vi "Update Map File Path.vi"(8 "error in (no error)":errorcluster, 10 "Map File Path":path, 11 "Map Model in":refnum<class "Map Model.lvclass">) -> (0 "error out":errorcluster, 3 "Map Model out":refnum<class "Map Model.lvclass">)   [LabVIEW 2020, in "Map Model.lvlib" / "Map Model.lvclass"]
uses:
  Map Model.lvclass
  <vilib>/Utility/miscctls.llb/LVPointTypeDef.ctl
  Map Model.lvclass/Map Model.ctl
  Stack/Stack.lvclass
panel:
  # "NOTICE -- YOU MUST LEAVE THIS NOTICE IN PLACE.\n\nCopyright (c) 2017, LIANG LIU Shawn.Liu.cn@gmail.com\nAll rights reserved.\n\nRedistribution and use in source and binary forms, with or without modification, are permitted provided that the following conditions are met:\n-Redistributions of source code must retain the above copyright notice, this list of conditions and the following disclaimer.\n-Redistributions in binary form must reproduce the above copyright notice, this list of conditions and the following disclaimer in the documentation and/or other materials provided with the distribution.\n-Neither the name of the eLp nor the names of its contributors may be used to endorse or promote products derived from this software without specific prior written permission.\n\nTHIS SOFTWARE IS PROVIDED BY THE COPYRIGHT HOLDERS AND CONTRIBUTORS \"AS IS\" AND ANY EXPRESS OR IMPLIED WARRANTIES, INCLUDING, BUT NOT LIMITED TO, THE IMPLIED WARRANTIES OF MERCHANTABILITY AND FITNESS FOR A PARTICULAR PURPOSE ARE DISCLAIMED. IN NO EVENT SHALL THE COPYRIGHT HOLDER OR CONTRIBUTORS BE LIABLE FOR ANY DIRECT, INDIRECT, INCIDENTAL, SPECIAL, EXEMPLARY, OR CONSEQUENTIAL DAMAGES (INCLUDING, BUT NOT LIMITED TO, PROCUREMENT OF SUBSTITUTE GOODS OR SERVICES; LOSS OF USE, DATA, OR PROFITS; OR BUSINESS INTERRUPTION) HOWEVER CAUSED AND ON ANY THEORY OF LIABILITY, WHETHER IN CONTRACT, STRICT LIABILITY, OR TORT (INCLUDING NEGLIGENCE OR OTHERWISE) ARISING IN ANY WAY OUT OF THE USE OF THIS SOFTWARE, EVEN IF ADVISED OF THE POSSIBILITY OF SUCH DAMAGE."
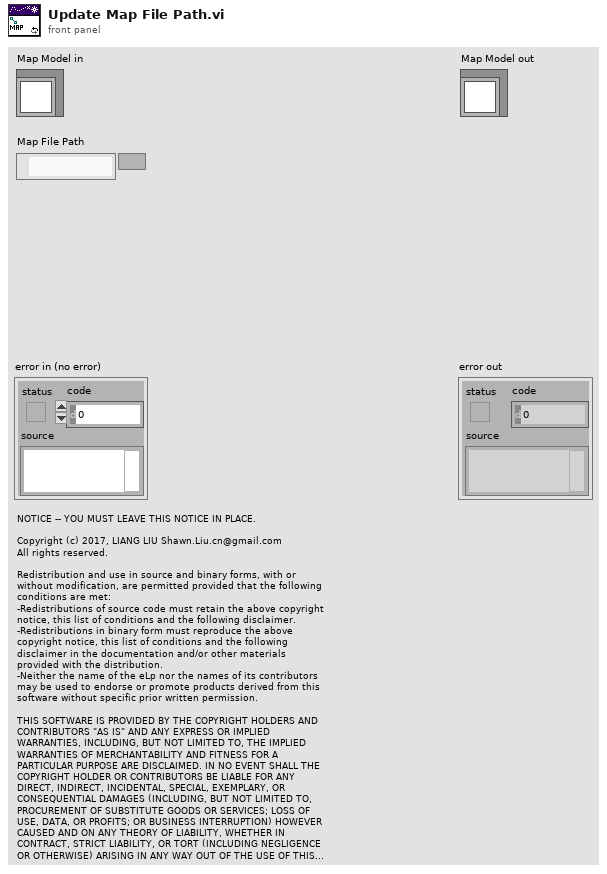
[diagram p1: front panel]
types:
  T1 = typedef "LVPointTypeDef.ctl" = cluster{"Horizontal":i16, "Vertical":i16}
  T2 = enum8{"Enabled", "Disabled", "Disabled and Grayed Out"}
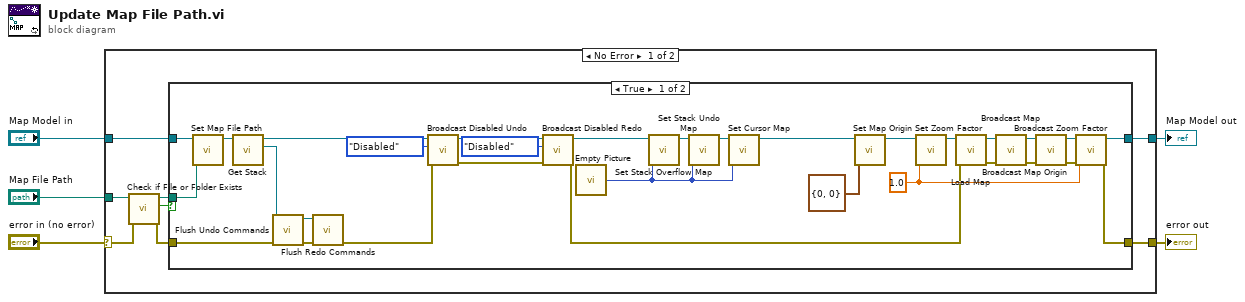
[diagram p0: block diagram]
diagram:
  n1 = case shown="No Error" "error in (no error)" {
    selector: "error in (no error)" -> [w9 w48]
    tunnel: "Map Model in" -> [w13 w47]
    tunnel: [w12 w48] -> w4
    tunnel: [w11 w47] -> w3
    tunnel: "Map File Path" -> [w10 _]
    frame No Error {
      n2 = call <vilib>:"Check if File or Folder Exists.vi"("error in (no error)"=w9, "path"=w10) -> ("error out"=w6:errorcluster, "file or folder exists?"=w7:bool, "dup path"=w8:path)  [unwired: 7 in]
      n3 = case shown="True" w7 {
        tunnel: w13 -> [w44 w46]
        tunnel: [w15 w45] -> w12
        tunnel: [w20 w46] -> w11
        tunnel: w8 -> [w43 _]
        tunnel: w6 -> [w27 w45]
        frame True {
          w19 = 1.0 ("Zoom Factor")
          n4 = call "Set Map File Path.vi"("Map File Path"=w43, "Map Model in"=w44) -> ("Map Model out"=w29:refnum<class "Map Model.lvclass">)  [unwired: 9 in]
          n5 = call "Get Stack.vi"("Map Model in"=w29) -> ("Stack"=w28:refnum<class "Stack.lvclass">, "Map Model out"=w32:refnum<class "Map Model.lvclass">)  [unwired: 9 in]
          n6 = call "Flush Undo Commands.vi"("error in (no error)"=w27, "Stack in"=w28) -> ("error out"=w37:errorcluster, "Stack out"=w36:refnum<class "Stack.lvclass">)  [unwired: 8 in]
          n7 = call "Flush Redo Commands.vi"("error in (no error)"=w37, "Stack in"=w36) -> ("error out"=w30:errorcluster)  [unwired: 8 in, 1 out]
          n8 = call "Broadcast Disabled Undo.vi"("error in (no error)"=w30, "Disabled Undo"=T2."Disabled", "Map Model in"=w32) -> ("error out"=w31:errorcluster, "Map Model out"=w35:refnum<class "Map Model.lvclass">)  [unwired: 7 in]
          n9 = call "Broadcast Disabled Redo.vi"("error in (no error)"=w31, "Disabled Redo"=T2."Disabled", "Map Model in"=w35) -> ("error out"=w18:errorcluster, "Map Model out"=w14:refnum<class "Map Model.lvclass">)  [unwired: 7 in]
          n10 = call "Empty Picture"() -> ("empty picture"=w38:picture)
          n11 = call "Set Stack Overflow Map.vi"("Stack Overflow Map"=w38, "Map Model in"=w14) -> ("Map Model out"=w40:refnum<class "Map Model.lvclass">)  [unwired: 9 in]
          n12 = call "Set Stack Undo Map.vi"("Stack Undo Map"=w38, "Map Model in"=w40) -> ("Map Model out"=w39:refnum<class "Map Model.lvclass">)  [unwired: 9 in]
          n13 = call "Set Cursor Map.vi"("Cursor Map"=w38, "Map Model in"=w39) -> ("Map Model out"=w26:refnum<class "Map Model.lvclass">)  [unwired: 9 in]
          n14 = call "Set Map Origin.vi"("Map Origin"=T1 {"Horizontal"=0, "Vertical"=0}, "Map Model in"=w26) -> ("Map Model out"=w25:refnum<class "Map Model.lvclass">)  [unwired: 9 in]
          n15 = call "Set Zoom Factor.vi"("Zoom Factor"=w19, "Map Model in"=w25) -> ("Map Model out"=w24:refnum<class "Map Model.lvclass">)  [unwired: 9 in]
          n16 = call "Load Map.vi"("error in (no error)"=w18, "Map Model in"=w24) -> ("error out"=w41:errorcluster, "Map Model out"=w42:refnum<class "Map Model.lvclass">)  [unwired: 8 in]
          n17 = call "Broadcast Map.vi"("error in (no error)"=w41, "Map Model in"=w42) -> ("error out"=w17:errorcluster, "Map Model out"=w23:refnum<class "Map Model.lvclass">)  [unwired: 8 in]
          n18 = call "Broadcast Map Origin.vi"("error in (no error)"=w17, "Map Model in"=w23) -> ("error out"=w16:errorcluster, "Map Model out"=w22:refnum<class "Map Model.lvclass">)  [unwired: 8 in]
          n19 = call "Broadcast Zoom Factor.vi"("error in (no error)"=w16, "Zoom Factor"=w19, "Map Model in"=w22) -> ("error out"=w15:errorcluster, "Map Model out"=w20:refnum<class "Map Model.lvclass">)  [unwired: 7 in]
        }
        frame False {
        }
      }
    }
    frame Error {
    }
  }
  "error out" <- w4
  "Map Model out" <- w3
